vi "PhotonVision_Aim_At_Target.vi"(6 "Y Axes":dbl, 8 "Init":bool, 9 "AprilTagID":i32, 10 "Use AprilTag":bool, 11 "CameraName":string) -> (1 "Right Motor Value":dbl, 3 "Left Motor Value":dbl)   [LabVIEW 2019]
uses:
  <vilib>/Rock Robotics/WPI/ThirdParty/PhotonVisionLib/PhotonVisionLib.lvlib
  <vilib>/Rock Robotics/WPI/Joystick/WPI_JoystickArcadeMapping.vi
  <vilib>/Rock Robotics/WPI/ThirdParty/JAS_Junk/TrajLib/Trajectory_Library.lvlib
  <vilib>/Rock Robotics/Network Tables/NT Write Number.vi
  <vilib>/Rock Robotics/Network Tables/NT Write Boolean.vi
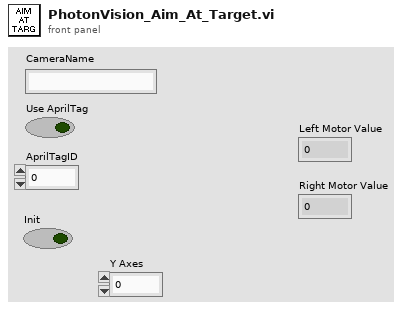
[diagram p1: front panel]
types:
  T1 = typedef "PhotonVisionLib.lvlib/PhotonPipelineResultType.ctl" = cluster{"Targets":T2[], "PhotonMultiTargetPNPResult":T8, "PhotonPipelineMetadata":T10}
  T2 = typedef "PhotonVisionLib.lvlib/PhotonTrackedTargetType.ctl" = cluster{"Yaw":dbl, "Pitch":dbl, "Area":dbl, "Skew":dbl, "MinAreaRectCorners":T3[], "BestCameraToTarget":T4, "FiducialId":i32, "AltCameraToTarget":T4, "PoseAmbiguity":dbl, "DetectedCorners":T3[], "ObjDetectId":i32, "ObjDetectConf":sgl}
  T3 = typedef "PhotonVisionLib.lvlib/TargetCornerType.ctl" = cluster{"X":dbl, "Y":dbl}
  T4 = typedef "Trajectory_Library.lvlib/TRANSFORM3D.ctl" = cluster{"TRANSLATION3D":T5, "ROTATION3D":T6, "XF":bool}
  T5 = typedef "Trajectory_Library.lvlib/TRANSLATION3D.ctl" = cluster{"X":dbl, "Y":dbl, "Z":dbl}
  T6 = typedef "Trajectory_Library.lvlib/ROTATION3D.ctl" = cluster{"Q_quaternion":T7}
  T7 = typedef "Trajectory_Library.lvlib/QUATERNION.ctl" = cluster{"R":dbl, "V":dbl[]}
  T8 = typedef "PhotonVisionLib.lvlib/PhotonMultiTargetPNPResultType.ctl" = cluster{"PhotonPNPResult":T9, "FiducialIDsUsed":i16[]}
  T9 = typedef "PhotonVisionLib.lvlib/PhotonPNPResultType.ctl" = cluster{"IsPresent":bool, "bestReprojErr":dbl, "altReprojErr":dbl, "ambiguity":dbl, "Best":T4, "Alt":T4}
  T10 = typedef "PhotonVisionLib.lvlib/PhotonPipelineMetadataType.ctl" = cluster{"CaptureTimestampMicros":i64, "PublishTimestampMicros":i64, "SequenceID":i64, "TimeSinceLastPong":i64}
  T11 = typedef "Trajectory_Library.lvlib/PID_ADV_LIMITS.ctl" = cluster{"MaxInput":dbl, "MinInput":dbl, "Continuous":bool, "MaxOutput":dbl, "MinOutput":dbl}
  T12 = typedef "Trajectory_Library.lvlib/PID_ADV_TUNING.ctl" = cluster{"Kf":dbl, "Kp":dbl, "Ki":dbl, "Kd":dbl, "MaximumIntegral":dbl, "MinimumIntegral":dbl, "Filter Derivative":bool, "IntegralZone":dbl}
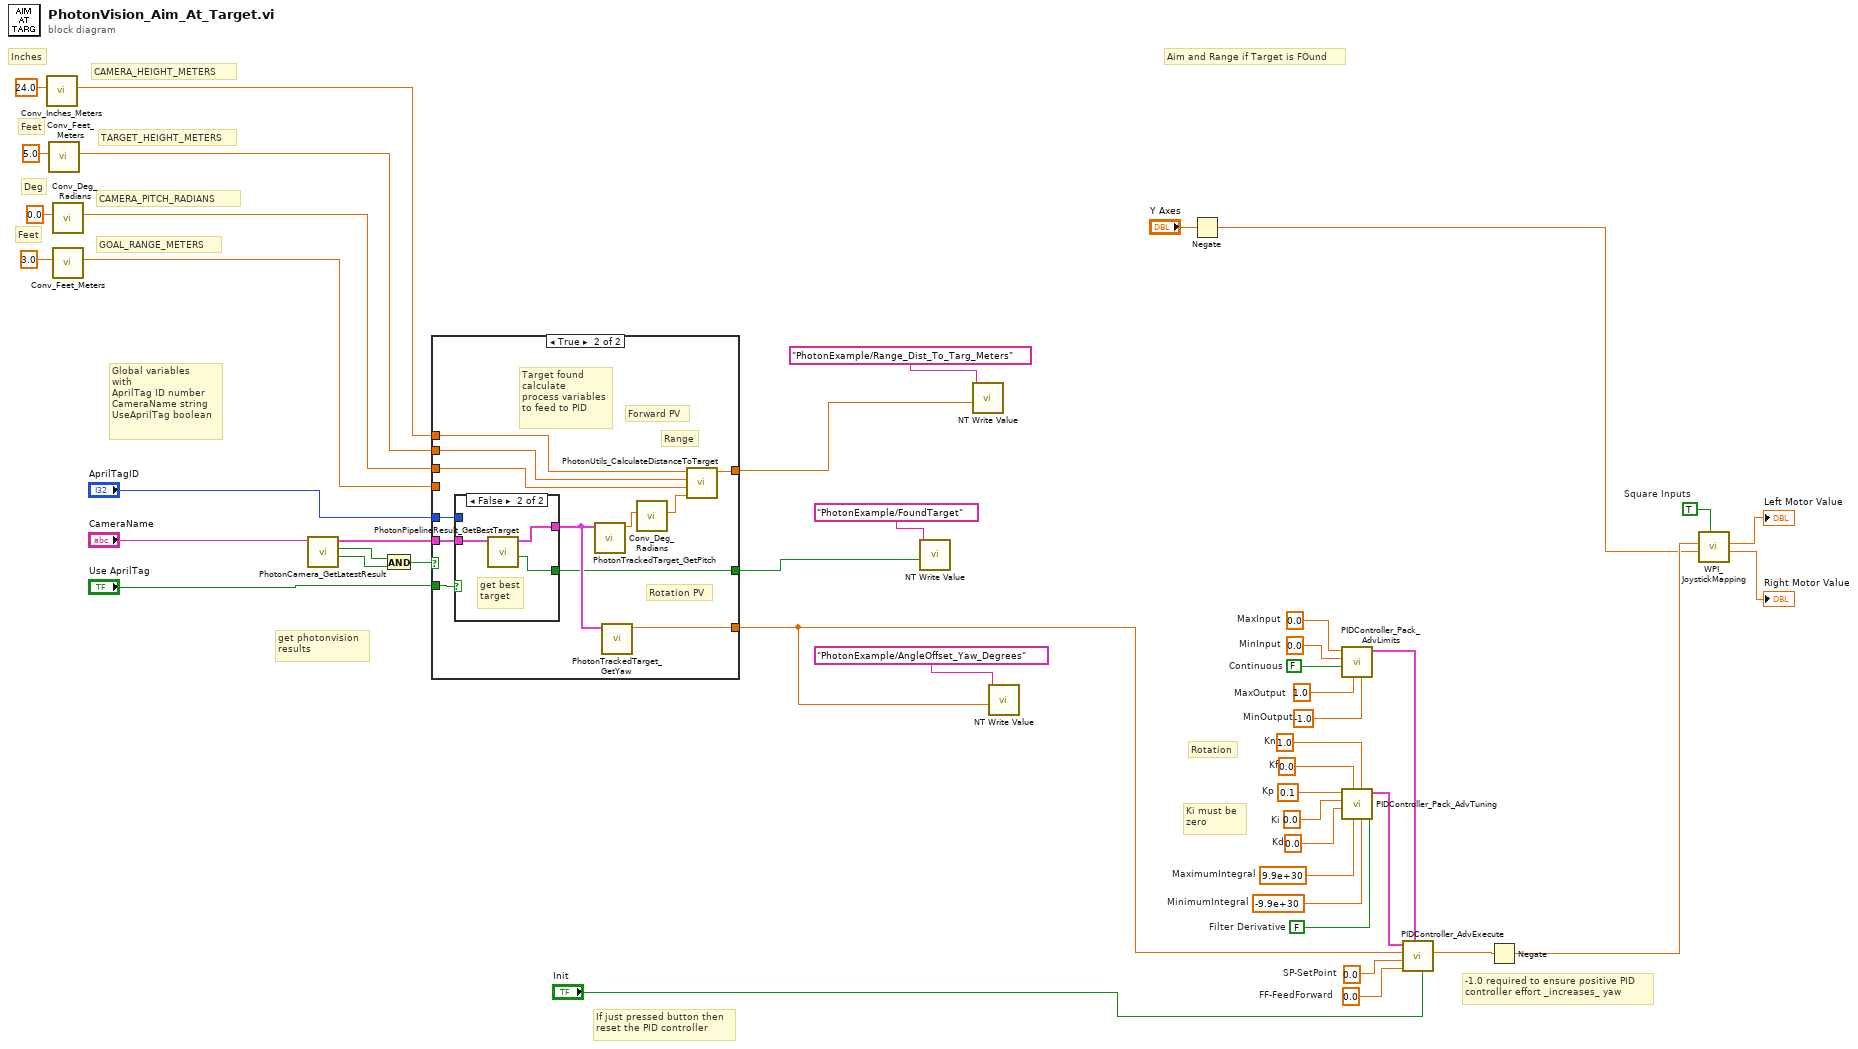
[diagram p0: block diagram]
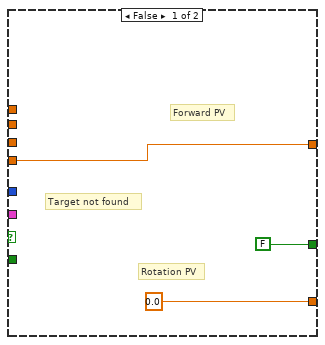
[diagram p2: hidden frame]
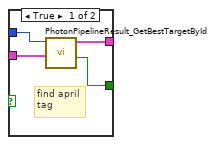
[diagram p3: hidden frame]
diagram:
  w33 = 0.0  # FF-FeedForward
  w31 = 0.0  # SP-SetPoint
  w15 = 1.0  # Kn
  w16 = 0.1  # Kp
  w17 = 0.0  # Ki
  w18 = 0.0  # Kd
  w19 = 0.0  # Kf
  w20 = 9.9e+30  # MaximumIntegral
  w21 = -9.9e+30  # MinimumIntegral
  w22 = FALSE  # Filter Derivative
  w24 = 0.0  # MinInput
  w25 = FALSE  # Continuous
  w26 = 1.0  # MaxOutput
  w23 = -1.0  # MinOutput
  w27 = 0.0  # MaxInput
  w12 = TRUE  # Square Inputs
  # "Global variables\nwith \nAprilTag ID number\nCameraName string\nUseAprilTag boolean"
  # "Feet"
  # "Deg"
  # "Feet"
  # "Inches"
  # "GOAL_RANGE_METERS"
  # "CAMERA_PITCH_RADIANS"
  # "TARGET_HEIGHT_METERS"
  # "CAMERA_HEIGHT_METERS"
  # "Aim and Range if Target is FOund"
  # "-1.0 required to ensure positive PID \ncontroller effort _increases_ yaw"
  # "Ki must be \nzero"
  # "If just pressed button then\nreset the PID controller"
  # "Rotation"
  # "get photonvision\nresults"
  n1 = call <vilib>:"Conv_Inches_Meters.vi"("INCH"=24.0) -> ("Meters"=w46:dbl)  [unwired: 10 in]
  n2 = call <vilib>:"Conv_Feet_Meters.vi"("Feet"=5.0) -> ("Meters"=w45:dbl)  [unwired: 10 in]
  n3 = call <vilib>:"Conv_Deg_Radians.vi"("Degress"=0.0) -> ("Radians"=w44:dbl)  [unwired: 10 in]
  n4 = call <vilib>:"Conv_Feet_Meters.vi"("Feet"=3.0) -> ("Meters"=w43:dbl)  [unwired: 10 in]
  n5 = call <vilib>:"PhotonCamera_GetLatestResult.vi"("CameraName"="CameraName") -> ("New Data"=w1:bool, "HasTargets"=w2:bool, "PipelineResult"=w30:T1)  [unwired: 6 in, 2 out]
  n6 = And(x=w2, y=w1) -> (x .and. y?=w3:bool)
  n7 = case shown="True" w3 {
    tunnel: w30 -> [_ w61]
    tunnel: [w48 w57] -> w5
    tunnel: [0.0 w56] -> w7
    tunnel: w46 -> [_ w53]
    tunnel: w45 -> [_ w54]
    tunnel: w44 -> [_ w55]
    tunnel: w43 -> [w48 _]
    tunnel: "Use AprilTag" -> [_ w52]
    tunnel: [FALSE ("TargetFound") w51] -> w38
    tunnel: "AprilTagID" -> [_ w50]
    frame False {
      # "Forward PV"
      # "Rotation PV"
      # "Target not found"
    }
    frame True {
      # "Target found\ncalculate\nprocess variables\nto feed to PID"
      # "Range"
      # "Forward PV"
      # "Rotation PV"
      n8 = case shown="False" w52 {
        tunnel: w61 -> [w63 w68]
        tunnel: [w65 w67] -> w58
        tunnel: [w64 w66] -> w51
        tunnel: w50 -> [w62 _]
        frame True {
          # "find april\ntag"
          n9 = call <vilib>:"PhotonPipelineResult_GetBestTargetById.vi"("PhotonPipelineResult"=w63, "FiducialId"=w62) -> ("Target Found"=w64:bool, "PhotonTrackedTarget"=w65:T2)  [unwired: 7 in, 1 out]
        }
        frame False {
          # "get best\ntarget"
          n10 = call <vilib>:"PhotonPipelineResult_GetBestTarget.vi"("PhotonPipelineResult"=w68) -> ("TargetFound"=w66:bool, "PhotonTrackedTarget"=w67:T2)  [unwired: 9 in]
        }
      }
      n11 = call <vilib>:"PhotonTrackedTarget_GetPitch.vi"("TrackedTarget"=w58) -> ("Pitch"=w60:dbl)  [unwired: 10 in]
      n12 = call <vilib>:"PhotonTrackedTarget_GetYaw.vi"("TrackedTarget"=w58) -> ("Yaw"=w56:dbl)  [unwired: 10 in]
      n13 = call <vilib>:"Conv_Deg_Radians.vi"("Degress"=w60) -> ("Radians"=w59:dbl)  [unwired: 10 in]
      n14 = call <vilib>:"PhotonUtils_CalculateDistanceToTarget.vi"("TargetPitch_Radians"=w59, "CameraPitch_Radians"=w55, "TargetHeight_Meters"=w54, "CameraHeight_Meters"=w53) -> ("DistanceToTarget_Meters"=w57:dbl)  [unwired: 7 in]
    }
  }
  n15 = call-poly <vilib>:"NT Write Value.vi"("value"=w38, "name"="PhotonExample/FoundTarget" ("Name")) -> ()  [unwired: 9 in, 1 out]
  n16 = call-poly <vilib>:"NT Write Value.vi"("value"=w5, "name"="PhotonExample/Range_Dist_To_Targ_Meters" ("Name")) -> ()  [unwired: 9 in, 1 out]
  n17 = call-poly <vilib>:"NT Write Value.vi"("value"=w7, "name"="PhotonExample/AngleOffset_Yaw_Degrees" ("Name")) -> ()  [unwired: 9 in, 1 out]
  n18 = Negate(x="Y Axes") -> (-x=w34:dbl)
  n19 = call <vilib>:"PIDController_Pack_AdvLimits.vi"("MinOutput"=w23, "MaxOutput"=w26, "Continuous"=w25, "MinInput"=w24, "MaxInput"=w27) -> ("Adv PID Limits"=w29:T11)  [unwired: 6 in]
  n20 = call <vilib>:"PIDController_Pack_AdvTuning.vi"("Filter Derivative"=w22, "MinimumIntegral"=w21, "Kn"=w15, "MaximumIntegral"=w20, "Kf"=w19, "Kd"=w18, "Ki"=w17, "Kp"=w16) -> ("Adv PID Tuning"=w28:T12)  [unwired: 3 in]
  n21 = call <vilib>:"PIDController_AdvExecute.vi"("Reset"="Init", "Adv PID Limits"=w29, "FF-FeedForward"=w33, "SP-SetPoint"=w31, "PV-Measurement"=w7, "Adv PID Tuning"=w28) -> ("CO-ControlOutput"=w35:dbl)  [unwired: 3 in, 2 out]
  n22 = Negate(x=w35) -> (-x=w36:dbl)
  n23 = call-poly <vilib>:"WPI_JoystickMapping.vi"("Square Inputs"=w12, "Y axis value"=w34, "X axis value"=w36) -> ("Right Motor Value"=→"Right Motor Value":dbl, "Left Motor Value"=→"Left Motor Value":dbl)  [unwired: 7 in]
